vi "test_ycar.vi"() -> ()   [LabVIEW 2019]
panel:
  in  "stop":bool
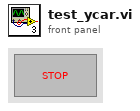
[diagram p1: front panel]
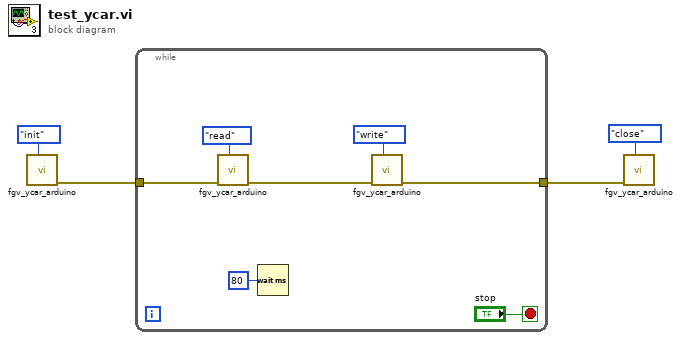
[diagram p0: block diagram]
diagram:
  n1 = call "fgv_ycar_arduino.vi"("cmd"=enum16{"init", "read", "write", "close"}."init") -> ("error out"=w3:errorcluster)  [unwired: 9 in, 1 out]
  n2 = while {
    tunnel: w3 -> [w8]
    tunnel: [w6] -> w1
    stop <- "stop" stop-if-true
    n3 = call "fgv_ycar_arduino.vi"("cmd"=enum16{"init", "read", "write", "close"}."read", "error in"=w8) -> ("error out"=w7:errorcluster)  [unwired: 8 in, 1 out]
    n4 = Wait (ms)(milliseconds to wait=u32 80) -> ()  [unwired: 1 out]
    n5 = call "fgv_ycar_arduino.vi"("cmd"=enum16{"init", "read", "write", "close"}."write", "error in"=w7) -> ("error out"=w6:errorcluster)  [unwired: 8 in, 1 out]
  }
  n6 = call "fgv_ycar_arduino.vi"("cmd"=enum16{"init", "read", "write", "close"}."close", "error in"=w1) -> ()  [unwired: 8 in, 2 out]
